vi "CovertGlobalto4Points.vi"(11 "Global Rectangle":i32[](array[numeric])) -> (3 "Array":string[](array[string]))   [LabVIEW 2019]
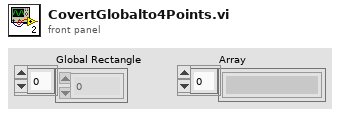
[diagram p1: front panel]
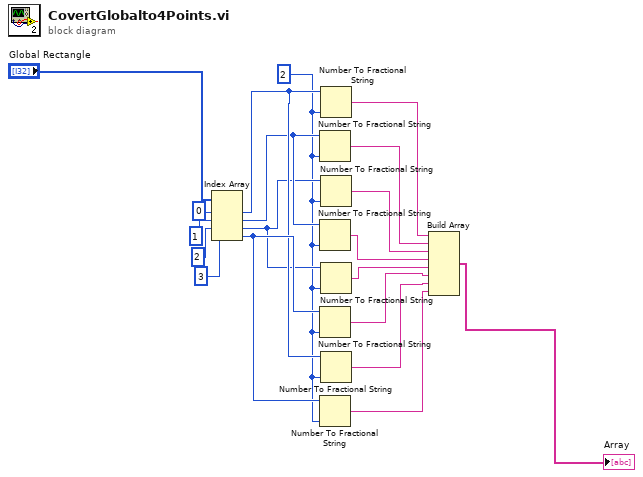
[diagram p0: block diagram]
diagram:
  w9 = i16 2 ("precision (6)")
  n1 = Index Array(array="Global Rectangle", index #1=0, index #2=1, index #3=2, index #4=3) -> (element #1=w12:i32, element #2=w11:i32, element #3=w10:i32, element #4=w13:i32)
  n2 = Number To Fractional String(number=w11, precision (6)=w9) -> (F-format string=w8:string)  [unwired: 2 in]
  n3 = Number To Fractional String(number=w11, precision (6)=w9) -> (F-format string=w15:string)  [unwired: 2 in]
  n4 = Number To Fractional String(number=w13, precision (6)=w9) -> (F-format string=w17:string)  [unwired: 2 in]
  n5 = Number To Fractional String(number=w13, precision (6)=w9) -> (F-format string=w19:string)  [unwired: 2 in]
  n6 = Number To Fractional String(number=w12, precision (6)=w9) -> (F-format string=w6:string)  [unwired: 2 in]
  n7 = Number To Fractional String(number=w10, precision (6)=w9) -> (F-format string=w14:string)  [unwired: 2 in]
  n8 = Number To Fractional String(number=w10, precision (6)=w9) -> (F-format string=w16:string)  [unwired: 2 in]
  n9 = Number To Fractional String(number=w12, precision (6)=w9) -> (F-format string=w18:string)  [unwired: 2 in]
  n10 = Build Array(w6, w8, w14, w15, w16, w17, w18, w19) -> (→"Array":string[])
